vi "CTL_SpecCheckLogic.vi"(7 "Drain!Fill In":bool, 8 "Level in":dbl, 9 "Spec Hi(n+1)":dbl, 10 "Spec Lo (n)":dbl, 11 "Spec Hi (n)":dbl) -> (0 "Vaild R?":bool, 1 "Measure R?":bool, 2 "Switch Range?":bool, 3 "In Range?":bool, 4 "Set Point":dbl)   [LabVIEW 2024]
panel:
  # "FILL LOGIC\nIn Range =    Spec Hi (n+1)  > Level > Spec Lo (n) \nSwitch Range =  Spec Hi (n) > Level > Spec Lo (n)\nMeausre R =  Level = {Spec Hi (n)  + Spec Hi (n+1)}/2 +/- 0.01 \nValid R = Spec Hi (n+1) > Level > Spec Hi (n)\n\nDRAIN LOGIC\nIn Range =  Spec Hi (n) > Level > Spec Hi (n+1)\nSwitch Range =  Spec Hi (n) > Level > Spec Lo (n)\nMeausre R =  Level = {Spec Lo (n)  + Spec Lo (n)}/2 +/- 0.01 \nValid R = Spec Lo (n) > Level > Spec Hi (n+1)"
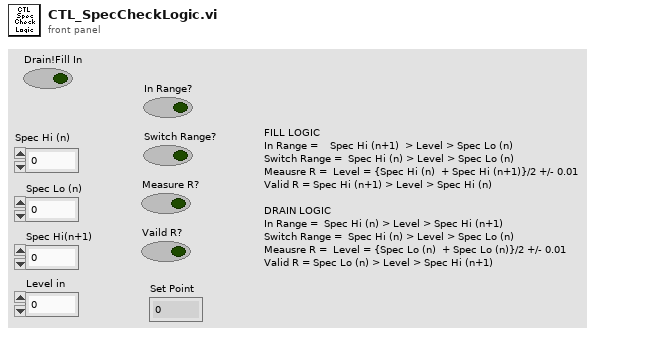
[diagram p1: front panel]
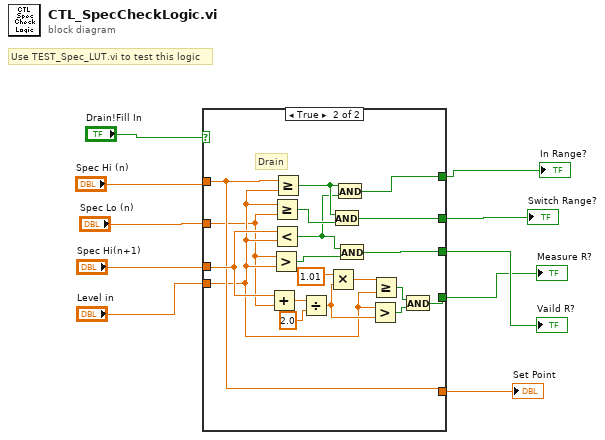
[diagram p0: block diagram]
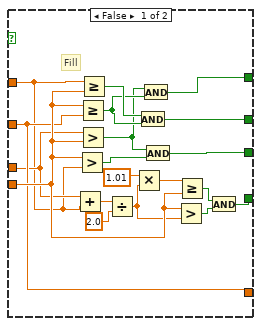
[diagram p2: hidden frame]
diagram:
  # "Use TEST_Spec_LUT.vi to test this logic"
  n1 = case shown="True" "Drain!Fill In" {
    tunnel: "Level in" -> [w18 w32]
    tunnel: "Spec Hi (n)" -> [w13 w36]
    tunnel: "Spec Hi(n+1)" -> [w14 w37]
    tunnel: [w29 w48] -> w5
    tunnel: "Spec Lo (n)" -> [w15 w30]
    tunnel: [w27 w47] -> w3
    tunnel: [w25 w46] -> w4
    tunnel: [w17 w39] -> w2
    tunnel: [w15 w36] -> w1
    frame False {
      # "Fill"
      n2 = Add(x=w14, y=w13) -> (x+y=w24:dbl)
      n3 = Greater?(x=w18, y=w13) -> (0:w28:bool)
      n4 = Greater Or Equal?(x=w18, y=w15) -> (x >= y?=w12:bool)
      n5 = Greater?(x=w14, y=w18) -> (0:w11:bool)
      n6 = Greater Or Equal?(x=w13, y=w18) -> (x >= y?=w26:bool)
      n7 = Divide(x=w24, y=2.0) -> (x/y=w16:dbl)
      n8 = Multiply(x=1.01, y=w16) -> (x*y=w19:dbl)
      n9 = And(x=w26, y=w12) -> (x .and. y?=w25:bool)
      n10 = And(x=w11, y=w12) -> (x .and. y?=w29:bool)
      n11 = And(x=w11, y=w28) -> (x .and. y?=w27:bool)
      n12 = Greater?(x=w18, y=w16) -> (0:w22:bool)
      n13 = Greater Or Equal?(x=w19, y=w18) -> (x >= y?=w21:bool)
      n14 = And(x=w21, y=w22) -> (x .and. y?=w17:bool)
    }
    frame True {
      # "Drain"
      n15 = Add(x=w37, y=w30) -> (x+y=w45:dbl)
      n16 = Greater?(x=w30, y=w32) -> (0:w31:bool)
      n17 = Greater Or Equal?(x=w32, y=w30) -> (x >= y?=w34:bool)
      n18 = Less?(x=w37, y=w32) -> (x < y?=w33:bool)
      n19 = Greater Or Equal?(x=w36, y=w32) -> (x >= y?=w35:bool)
      n20 = Divide(x=w45, y=2.0) -> (x/y=w38:dbl)
      n21 = Multiply(x=1.01, y=w38) -> (x*y=w40:dbl)
      n22 = And(x=w35, y=w34) -> (x .and. y?=w46:bool)
      n23 = And(x=w35, y=w33) -> (x .and. y?=w48:bool)
      n24 = And(x=w33, y=w31) -> (x .and. y?=w47:bool)
      n25 = Greater?(x=w32, y=w38) -> (0:w43:bool)
      n26 = Greater Or Equal?(x=w40, y=w32) -> (x >= y?=w42:bool)
      n27 = And(x=w42, y=w43) -> (x .and. y?=w39:bool)
    }
  }
  "In Range?" <- w5
  "Switch Range?" <- w4
  "Vaild R?" <- w3
  "Measure R?" <- w2
  "Set Point" <- w1
